vi "Modbus Slave Example.vi"() -> ()   [LabVIEW 2014, in "MyLib.lvlib"]
doc: "An example of the modbus master functionality."
uses:
  MyLib.lvlib
  Network Protocol/Network Slave/daemon status.ctl
  Network Protocol/Network Slave/TCP/Connection.ctl
  API/Slave/Modbus Slave.lvclass
  Data Model/Identification Parameters.ctl
  API/Wrapper/Create TCP Slave.vi
  API/Wrapper/API Main.lvlib
  Data Model/Device Data Model.lvclass
  Network Protocol/Network Slave/Network Slave.lvclass
  Network Protocol/Network Slave/TCP/TCP Slave.lvclass
panel:
  out "TCP Connection List":T1[](array[typedef])
  out "TCP Connection Count":u32
  out "Daemon Error":errorcluster
  out "Daemon Status":T2
  in  "Stop Button":bool
  in  "Port":u16=502
  in  "Fetch Holding Registers":bool
  in  "Fetch Coils":bool
  in  "Set Discrete Inputs":bool
  in  "Set Input Registers":bool
  in  "Set Basic Objects":bool
  in  "Basic Objects":string[](array[string])=["National Instruments", "42", "1.0.0"]
  out "Status":string
  out "Holding Registers":u16[](array[numeric])
  in  "Input Registers":u16[](array[numeric])=[0, 0, 0, 0, 0, 0, 0, 0]
  out "Coils":bool[](array[boolean])
  in  "Discrete Inputs":bool[](array[boolean])
  # "Holding Registers are the integer outputs of a modbus device. This example allows you to read the first 8 outputs."
  # "Coils are the boolean outputs of a modbus device. This example allows you to read the first 8 outputs."
  # "Modbus devices can also store objects in their memory, which are variable length strings. This example sets the basic level of objects."
  # "Discrete inputs are the boolean inputs of a modbus device. This example allows you to set the first 8 inputs."
  # "Input Registers are the integer inputs of a modbus device. This example allows you to set the first 8 inputs."
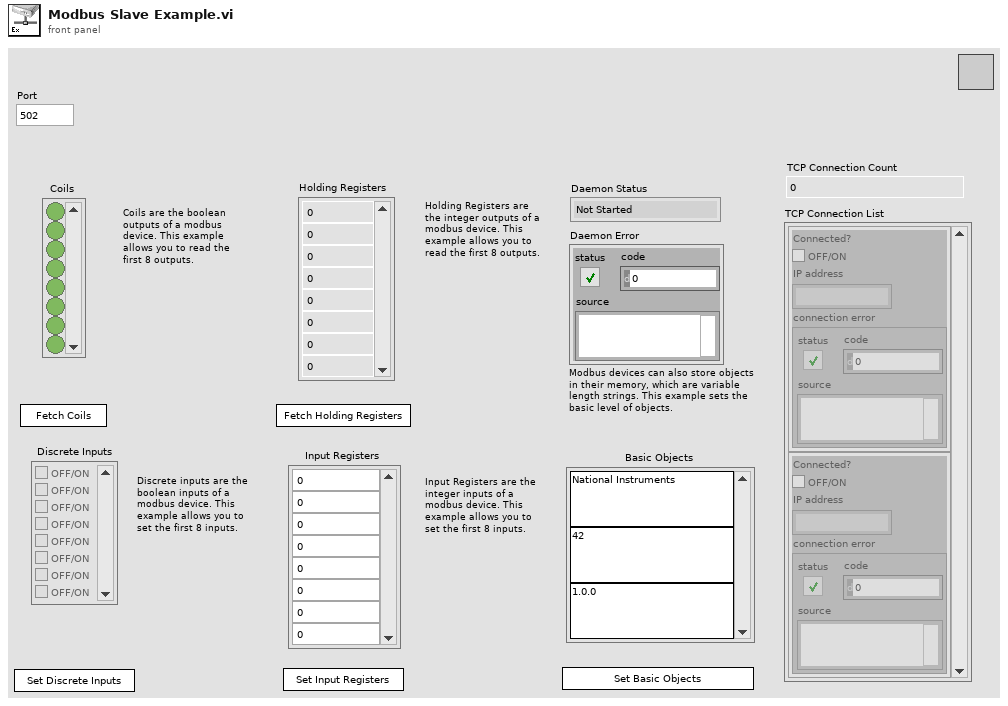
[diagram p1: front panel]
types:
  T1 = typedef "MyLib.lvlib/TCP Slave.lvclass/Connection.ctl" = cluster{"Connected?":bool, "IP address":string, "connection error":errorcluster}
  T2 = typedef "MyLib.lvlib/Network Slave.lvclass/daemon status.ctl" = enum16{"Not Started", "Running", "Error", "Stopped"}
  T3 = typedef "MyLib.lvlib/Device Data Model.lvclass/Identification Parameters.ctl" = cluster{"Object ID":u8, "Value":string}
  T4 = typedef "Network Slave.lvclass/daemon status.ctl" = enum16{"Not Started", "Running", "Error", "Stopped"}
  T5 = typedef "TCP Slave.lvclass/Connection.ctl" = cluster{"Connected?":bool, "IP address":string, "connection error":errorcluster}
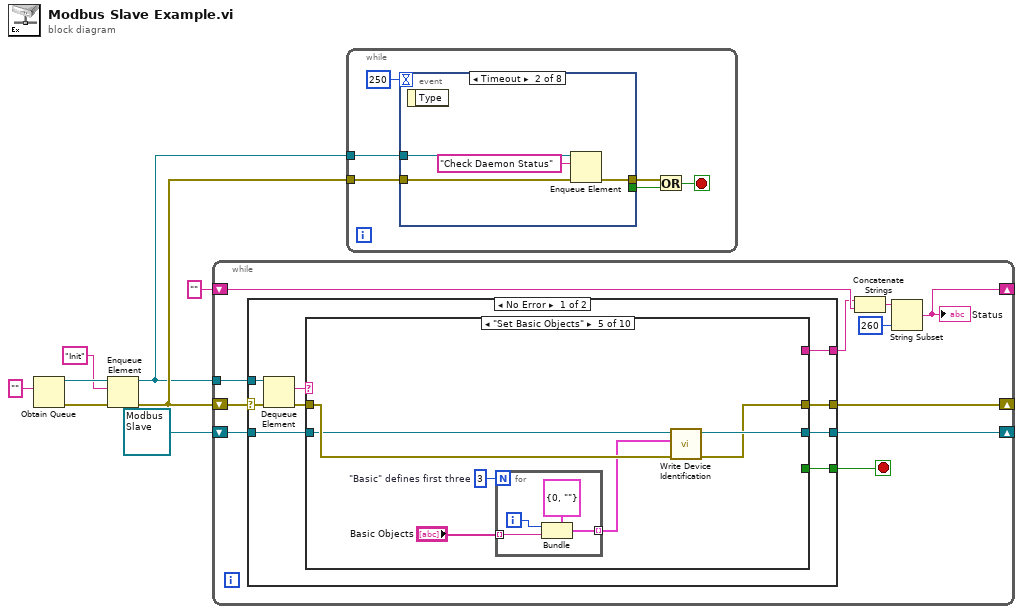
[diagram p0: block diagram]
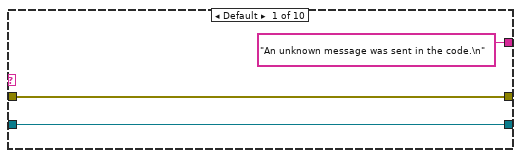
[diagram p2: hidden frame]
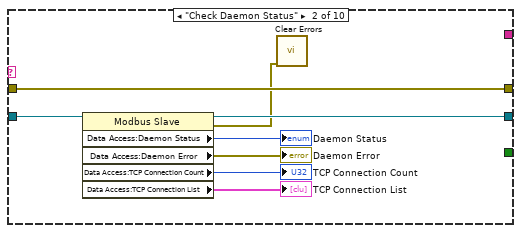
[diagram p3: hidden frame]
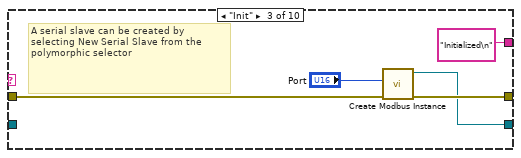
[diagram p4: hidden frame]
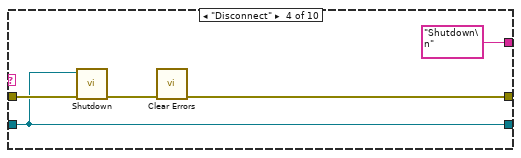
[diagram p5: hidden frame]
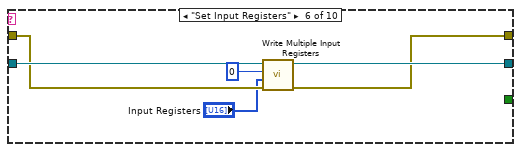
[diagram p6: hidden frame]
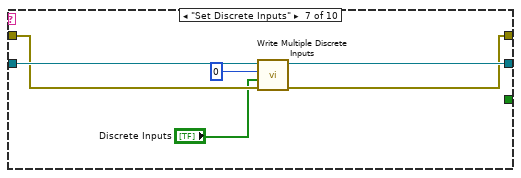
[diagram p7: hidden frame]
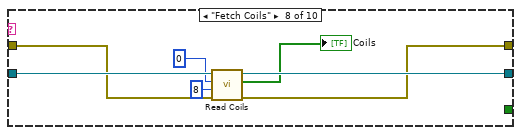
[diagram p8: hidden frame]
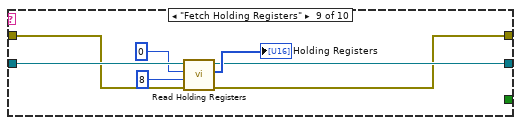
[diagram p9: hidden frame]
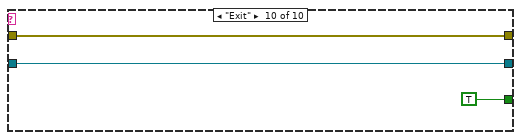
[diagram p10: hidden frame]
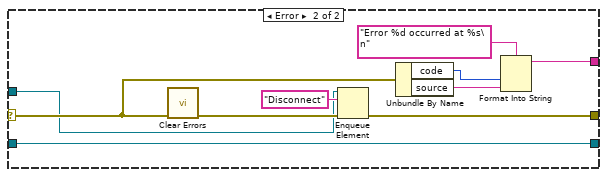
[diagram p11: hidden frame]
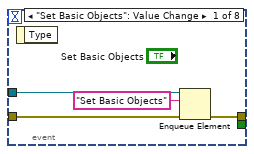
[diagram p12: hidden frame]
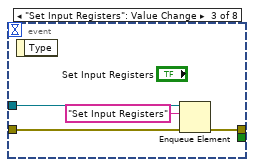
[diagram p13: hidden frame]
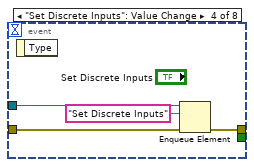
[diagram p14: hidden frame]
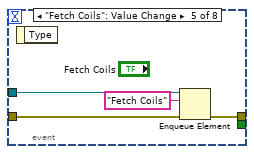
[diagram p15: hidden frame]
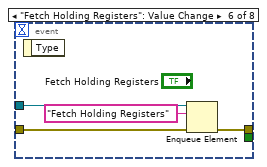
[diagram p16: hidden frame]
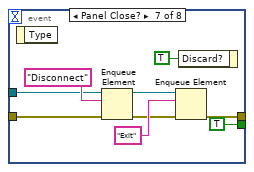
[diagram p17: hidden frame]
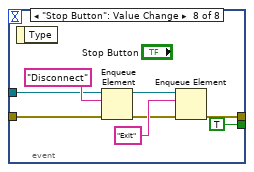
[diagram p18: hidden frame]
diagram:
  n1 = Obtain Queue(element data type="") -> (queue out=w4:refnum<queue>, error out=w8:errorcluster)  [unwired: 4 in, 1 out]
  n2 = Enqueue Element(queue=w4, element="Init", error in (no error)=w8) -> (queue out=w3:refnum<queue>, error out=w5:errorcluster)  [unwired: 1 in, 1 out]
  n3 = while {
    shift-right: [w9] -> _
    shift-left: refnum<class "Modbus Slave.lvclass"> refnum ("Modbus Slave") -> [w12]
    tunnel: w3 -> [w19]
    shift-right: [w10] -> _
    shift-left: w5 -> [w18]
    shift-right: [w17] -> _
    shift-left: "" ("Status") -> [w14]
    stop <- w11 stop-if-true
    n4 = case shown="No Error" w18 {
      selector: w18 -> [w27 w97]
      tunnel: w19 -> [w28 w91]
      tunnel: [w24 w98] -> w10
      tunnel: [w21 w94] -> w13
      tunnel: [w23 w90] -> w9
      tunnel: w12 -> [w22 w90]
      tunnel: [w20 _] -> w11
      frame No Error {
        n5 = Dequeue Element(queue=w28, error in (no error)=w27) -> (element=w25:string, error out=w26:errorcluster)  [unwired: 1 in, 2 out]
        n6 = case shown="\"Set Basic Objects\"" w25 {
          tunnel: w26 -> [w31 w39 w44 w49 w56 w63 w69 w76 w85 w89]
          tunnel: [w31 w39 w43 w45 w51 w64 w70 w74 w82 w89] -> w24
          tunnel: [w30 w37 w42 w47 w55 w65 w71 w75 w83 w88] -> w23
          tunnel: w22 -> [w30 w38 _ w47 w54 w66 w72 w79 w86 w88]
          tunnel: ["An unknown message was sent in the code.\n" _ "Initialized\n" "Shutdown\n" _ _ _ _ _ _] -> w21
          tunnel: [_ _ _ _ _ _ _ _ _ TRUE] -> w20
          frame Default {
          }
          frame "Check Daemon Status" {
            n7 = property class="Modbus Slave"(reference=w38) -> (reference out=w37:refnum<class "Modbus Slave.lvclass">, error out=w36:errorcluster, "Data Access:Daemon Status"=→"Daemon Status":T4, "Data Access:Daemon Error"=→"Daemon Error":errorcluster, "Data Access:TCP Connection Count"=→"TCP Connection Count":u32, "Data Access:TCP Connection List"=→"TCP Connection List":T5[])  [unwired: 1 in]
            n8 = call <vilib>:"Clear Errors.vi"("error in (no error)"=w36) -> ()  [unwired: 5 in, 2 out]
          }
          frame "Init" {
            # "A serial slave can be created by selecting New Serial Slave from the polymorphic selector"
            n9 = call-poly "Create Modbus Instance.vi"("error in"=w44, "port (502)"="Port") -> ("error out"=w43:errorcluster, "TCP slave instance"=w42:refnum<class "Modbus Slave.lvclass">)  [unwired: 8 in]
          }
          frame "Disconnect" {
            n10 = call-dynamic "Shutdown.vi"("error in"=w49, "Modbus slave in"=w47) -> ("error out"=w48:errorcluster)  [unwired: 9 in]
            n11 = call <vilib>:"Clear Errors.vi"("error in (no error)"=w48) -> ("error out"=w45:errorcluster)  [unwired: 5 in, 1 out]
          }
          frame "Set Basic Objects" {
            w50 = 3  # "Basic" defines first three
            n12 = for {
              N: w50 -> [_]
              tunnel: "Basic Objects" -> [w58] mode=indexing
              tunnel: [w57] -> w52 mode=indexing
              i -> [w59]
              n13 = Bundle(cluster=T3 {"Object ID"=0, "Value"=""} ("Parameters"), "Object ID"=w59, "Value"=w58) -> (w57:T3)
            }
            n14 = call-dynamic "Write Device Identification.vi"("error in"=w56, "objects"=w52, "Modbus slave in"=w54) -> ("error out"=w51:errorcluster, "Modbus slave out"=w55:refnum<class "Modbus Slave.lvclass">)  [unwired: 7 in]
          }
          frame "Set Input Registers" {
            n15 = call-dynamic "Write Multiple Input Registers.vi"("error in"=w63, "input registers to write"="Input Registers", "starting address"=u16 0, "Modbus slave in"=w66) -> ("error out"=w64:errorcluster, "Modbus slave out"=w65:refnum<class "Modbus Slave.lvclass">)  [unwired: 6 in]
          }
          frame "Set Discrete Inputs" {
            n16 = call-dynamic "Write Multiple Discrete Inputs.vi"("error in"=w69, "discrete inputs to write"="Discrete Inputs", "starting address"=u16 0, "Modbus slave in"=w72) -> ("error out"=w70:errorcluster, "Modbus slave out"=w71:refnum<class "Modbus Slave.lvclass">)  [unwired: 6 in]
          }
          frame "Fetch Coils" {
            n17 = call-dynamic "Read Coils.vi"("error in"=w76, "number of inputs"=u16 8 ("number of coils"), "starting address"=u16 0, "Modbus slave in"=w79) -> ("error out"=w74:errorcluster, "coils"=→"Coils":bool[], "Modbus slave out"=w75:refnum<class "Modbus Slave.lvclass">)  [unwired: 5 in]
          }
          frame "Fetch Holding Registers" {
            n18 = call-dynamic "Read Holding Registers.vi"("error in"=w85, "number of inputs"=u16 8 ("number of registers"), "starting address"=u16 0, "Modbus slave in"=w86) -> ("error out"=w82:errorcluster, "register values"=→"Holding Registers":u16[], "Modbus slave out"=w83:refnum<class "Modbus Slave.lvclass">)  [unwired: 5 in]
          }
          frame "Exit" {
          }
        }
      }
      frame Error {
        n19 = call <vilib>:"Clear Errors.vi"("error in (no error)"=w97) -> ("error out"=w99:errorcluster)  [unwired: 5 in, 1 out]
        n20 = Enqueue Element(queue=w91, element="Disconnect", error in (no error)=w99) -> (error out=w98:errorcluster)  [unwired: 1 in, 2 out]
        n21 = Unbundle By Name(w97) -> ("code"=w96:i32, "source"=w95:string)
        n22 = Format Into String(format string="Error %d occurred at %s\n", w96, w95) -> (resulting string=w94:string)  [unwired: 2 in, 1 out]
      }
    }
    n23 = Concatenate Strings(w13, w14) -> (w15:string)
    n24 = String Subset(string=w15, length (rest)=260 ("length (rest)")) -> (substring=w17:string)  [unwired: 1 in]
    "Status" <- w17
  }
  n25 = while {
    tunnel: w5 -> [w105]
    tunnel: w3 -> [w104]
    stop <- w101 stop-if-true
    n26 = event shown="[1] Timeout" {
      selector: _ -> [_ _ _ _ _ _ _ _]
      dyn-events: _ -> [_ _ _ _ _ _ _ _]
      timeout: 250 -> [_ _ _ _ _ _ _ _]
      tunnel: w105 -> [w109 w113 w117 w121 w125 w129 w135 w144]
      tunnel: [w108 w112 w116 w120 w124 w128 w130 w139] -> w103
      tunnel: w104 -> [w107 w111 w115 w119 w123 w127 w132 w141]
      tunnel: [_ _ _ _ _ _ TRUE ("Discard?") TRUE ("Discard?")] -> w102
      event "Set Basic Objects": Value Change {
        n27 = event-data() -> ()  [unwired: 1 in, 1 out]
        n28 = Enqueue Element(queue=w107, element="Set Basic Objects", error in (no error)=w109) -> (error out=w108:errorcluster)  [unwired: 1 in, 2 out]
      }
      event Timeout {
        n29 = event-data() -> ()  [unwired: 1 in, 1 out]
        n30 = Enqueue Element(queue=w111, element="Check Daemon Status", error in (no error)=w113) -> (error out=w112:errorcluster)  [unwired: 1 in, 2 out]
      }
      event "Set Input Registers": Value Change {
        n31 = event-data() -> ()  [unwired: 1 in, 1 out]
        n32 = Enqueue Element(queue=w115, element="Set Input Registers", error in (no error)=w117) -> (error out=w116:errorcluster)  [unwired: 1 in, 2 out]
      }
      event "Set Discrete Inputs": Value Change {
        n33 = event-data() -> ()  [unwired: 1 in, 1 out]
        n34 = Enqueue Element(queue=w119, element="Set Discrete Inputs", error in (no error)=w121) -> (error out=w120:errorcluster)  [unwired: 1 in, 2 out]
      }
      event "Fetch Coils": Value Change {
        n35 = event-data() -> ()  [unwired: 1 in, 1 out]
        n36 = Enqueue Element(queue=w123, element="Fetch Coils", error in (no error)=w125) -> (error out=w124:errorcluster)  [unwired: 1 in, 2 out]
      }
      event "Fetch Holding Registers": Value Change {
        n37 = event-data() -> ()  [unwired: 1 in, 1 out]
        n38 = Enqueue Element(queue=w127, element="Fetch Holding Registers", error in (no error)=w129) -> (error out=w128:errorcluster)  [unwired: 1 in, 2 out]
      }
      event Panel Close? {
        n39 = event-data() -> ()  [unwired: 1 in, 1 out]
        n40 = Enqueue Element(queue=w132, element="Disconnect", error in (no error)=w135) -> (queue out=w133:refnum<queue>, error out=w131:errorcluster)  [unwired: 1 in, 1 out]
        n41 = Enqueue Element(queue=w133, element="Exit", error in (no error)=w131) -> (error out=w130:errorcluster)  [unwired: 1 in, 2 out]
        n42 = event-data("Discard?"=TRUE) -> ()  [unwired: 1 in, 1 out]
      }
      event "Stop Button": Value Change {
        n43 = event-data() -> ()  [unwired: 1 in, 1 out]
        n44 = Enqueue Element(queue=w141, element="Disconnect", error in (no error)=w144) -> (queue out=w142:refnum<queue>, error out=w140:errorcluster)  [unwired: 1 in, 1 out]
        n45 = Enqueue Element(queue=w142, element="Exit", error in (no error)=w140) -> (error out=w139:errorcluster)  [unwired: 1 in, 2 out]
      }
    }
    n46 = Or(x=w103, y=w102) -> (x .or. y?=w101:bool)
  }
